vi "Get status.vi"(8 "error in (no error)":errorcluster, 10 "motor ip":string) -> (0 "error out":errorcluster, 1 "error":bool, 2 "status":T1, 3 "mech_id":u8)   [LabVIEW 2018]
panel:
  in  "offline test":bool
  in  "response array":string[](array[string])
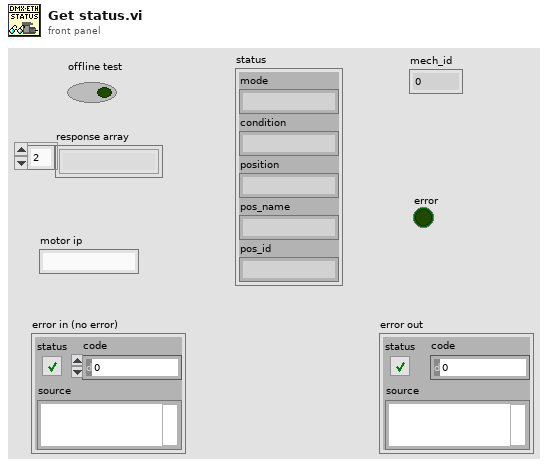
[diagram p1: front panel]
types:
  T1 = cluster{"mode":string, "condition":string, "position":string, "pos_name":string, "pos_id":string}
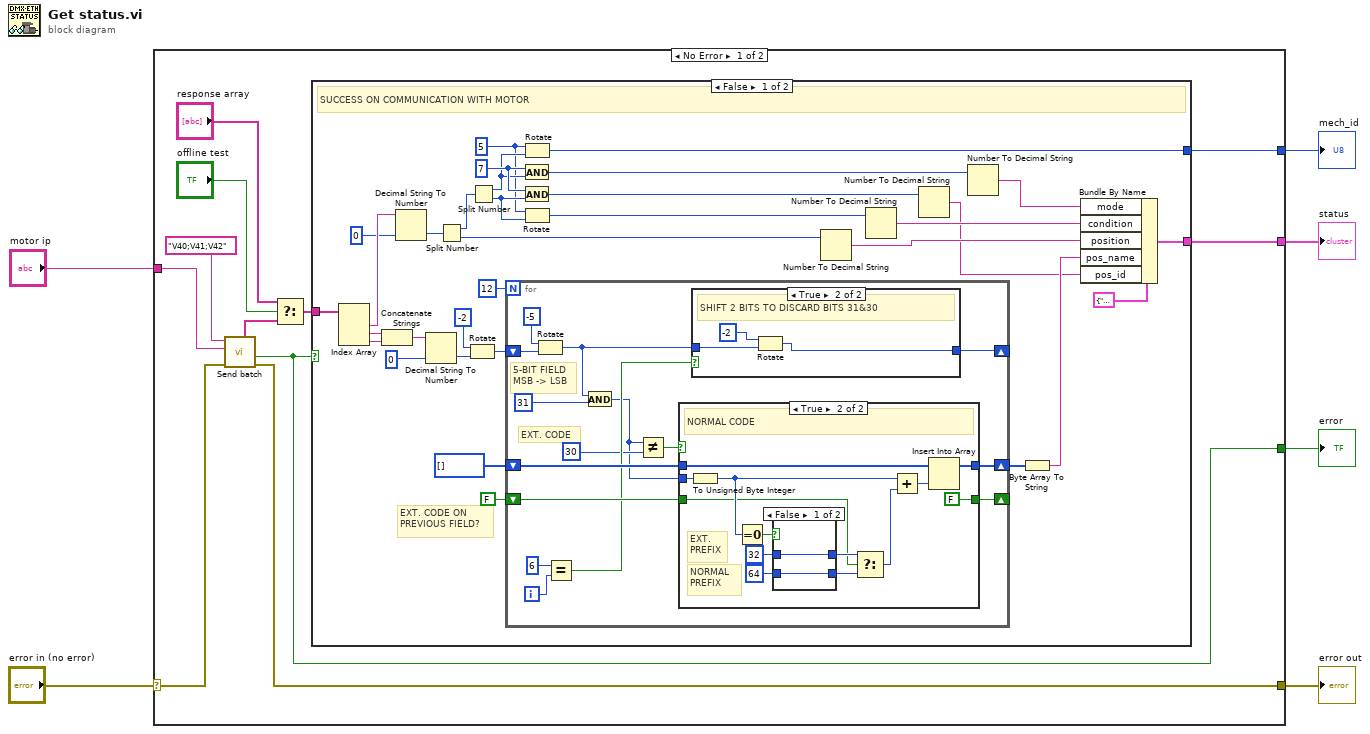
[diagram p0: block diagram]
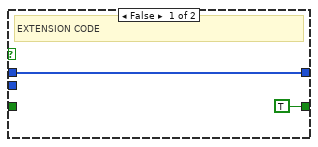
[diagram p3: hidden frame]
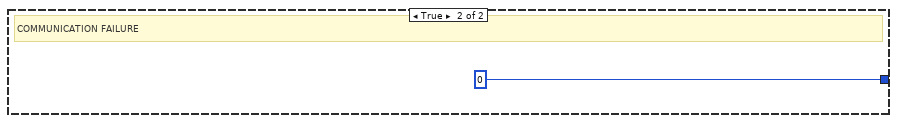
[diagram p5: hidden frame]
diagram:
  n1 = case shown="No Error" "error in (no error)" {
    selector: "error in (no error)" -> [w17 w89]
    tunnel: "motor ip" -> [w16 _]
    tunnel: [w14 _] -> w4
    tunnel: [w13 w89] -> w3
    tunnel: [w12 _] -> w2
    tunnel: [w11 _] -> w1
    frame No Error {
      n2 = call "Send batch.vi"("error in (no error)"=w17, "motor ip"=w16, "instruction"="V40;V41;V42") -> ("error out"=w13:errorcluster, "error"=w11:bool, "response array"=w9:string[])  [unwired: 4 in, 2 out]
      n3 = Select(t="response array", s="offline test", f=w9) -> (s? t:f=w10:string[])
      n4 = case shown="False" w11 {
        tunnel: w10 -> [w49 _]
        tunnel: [w41 u8 0] -> w14
        tunnel: [w18 _] -> w12
        frame False {
          w42 = u8 5 ("hi(x)")
          w45 = u8 7 ("hi(x)")
          # "EXT. CODE ON\nPREVIOUS FIELD?"
          # "SUCCESS ON COMMUNICATION WITH MOTOR"
          n5 = Index Array(array=w49) -> (element #1=w48:string, element #2=w38:string, element #3=w37:string)  [unwired: 3 in]
          n6 = Concatenate Strings(w38, w37) -> (w36:string)
          n7 = Decimal String To Number(string=w48, default (0L)=u32 0 ("default (0 I32)")) -> (number=w47:u32)  [unwired: 1 in, 1 out]
          n8 = Decimal String To Number(string=w36, default (0L)=u64 0 ("default (0 I32)")) -> (number=w34:u64)  [unwired: 1 in, 1 out]
          n9 = Split Number(x=w47) -> (hi(x)=w46:u16, lo(x)=w26:u16)
          n10 = Rotate(1:w34, 2:i16 -2 ("default (0 I32)")) -> (0:w32:u64)
          n11 = Split Number(x=w46) -> (hi(x)=w44:u8, lo(x)=w43:u8)
          n12 = for {
            N: 12 -> [_]
            shift-right: [w54] -> _
            shift-left: w32 -> [w63]
            shift-right: [w59] -> w29
            shift-left: u8[] [] ("constant") -> [w60]
            shift-right: [w58] -> _
            shift-left: FALSE -> [w61]
            i -> [w57]
            # "5-BIT FIELD\nMSB -> LSB"
            # "EXT. CODE"
            n13 = Rotate(1:w63, 2:i16 -5 ("hi(x)")) -> (0:w51:u64)
            n14 = Equal?(x=6, y=w57) -> (x = y?=w55:bool)
            n15 = And(x=w51, y=u64 31 ("hi(x)")) -> (x .and. y?=w52:u64)
            n16 = Not Equal?(x=w52, y=u64 30 ("hi(x)")) -> (x != y?=w62:bool)
            n17 = case shown="True" w62 {
              tunnel: w52 -> [_ w83]
              tunnel: w61 -> [_ w76]
              tunnel: w60 -> [w70 w73]
              tunnel: [w70 w72] -> w59
              tunnel: [TRUE FALSE] -> w58
              frame False {
                # "EXTENSION CODE"
              }
              frame True {
                # "NORMAL\nPREFIX"
                # "EXT. \nPREFIX"
                # "NORMAL CODE"
                n18 = To Unsigned Byte Integer(number=w83) -> (unsigned 8bit integer=w79:u8)
                n19 = Equal To 0?(x=w79) -> (x = 0?=w82:bool)
                n20 = case shown="False" w82 {
                  tunnel: u8 32 ("y") -> [w85 w86]
                  tunnel: u8 64 ("y") -> [w84 w87]
                  tunnel: [w85 w87] -> w78
                  tunnel: [w84 w86] -> w77
                  frame False {
                  }
                  frame True {
                  }
                }
                n21 = Select(t=w78, s=w76, f=w77) -> (s? t:f=w75:u8)
                n22 = Add(x=w79, y=w75) -> (x+y=w74:u8)
                n23 = Insert Into Array(array=w73, new element=w74) -> (w72:u8[])  [unwired: 1 in]
              }
            }
            n24 = case shown="True" w55 {
              tunnel: w51 -> [w65 w67]
              tunnel: [w65 w66] -> w54
              frame False {
              }
              frame True {
                # "SHIFT 2 BITS TO DISCARD BITS 31&30"
                n25 = Rotate(1:w67, 2:i16 -2 ("hi(x)")) -> (0:w66:u64)
              }
            }
          }
          n26 = Rotate(1:w44, 2:w42) -> (0:w41:u8)
          n27 = And(x=w45, y=w44) -> (x .and. y?=w20:u8)
          n28 = And(x=w45, y=w43) -> (x .and. y?=w22:u8)
          n29 = Rotate(1:w43, 2:w42) -> (0:w24:u8)
          n30 = Number To Decimal String(number=w26) -> (decimal integer string=w25:string)  [unwired: 1 in]
          n31 = Number To Decimal String(number=w24) -> (decimal integer string=w23:string)  [unwired: 1 in]
          n32 = Number To Decimal String(number=w22) -> (decimal integer string=w21:string)  [unwired: 1 in]
          n33 = Number To Decimal String(number=w20) -> (decimal integer string=w19:string)  [unwired: 1 in]
          n34 = Byte Array To String(unsigned byte array=w29) -> (string=w27:string)
          n35 = Bundle By Name(cluster=T1 {"mode"="", "condition"="", "position"="", "pos_name"="", "pos_id"=""} ("status"), "mode"=w19, "condition"=w23, "position"=w25, "pos_name"=w27, "pos_id"=w21) -> (w18:T1)
        }
        frame True {
          # "COMMUNICATION FAILURE"
        }
      }
    }
    frame Error {
    }
  }
  "mech_id" <- w4
  "error out" <- w3
  "status" <- w2
  "error" <- w1
